vi "Channels.vi"() -> (2 "Names":string[](array[string]), 3 "Channels to Create":T1[](array[typedef]) {"Custom Config Data" format="%x"})   [LabVIEW 2021, in "TemplateCommon.lvlib"]
uses:
  TemplateCommon.lvlib
  CIF-LVCore/src/Channels/ChannelRegistrar/typedef/Channel Definition.ctl
  <vilib>/CIF Foundation/CIF Channels Core/CIFChannels/Typedef/Direction.ctl
  CIF-LVCore/src/Channels/ChannelRegistrar/typedef/Registered Channel Types.ctl
  CIF-LVCore/src/Channels/ChannelRegistrar/ChannelRegistrar.lvlib
  <vilib>/CIF Foundation/CIF Channels Core/CIFChannels/CIFChannels.lvclass
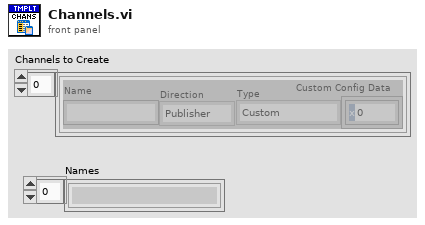
[diagram p1: front panel]
types:
  T1 = typedef "ChannelRegistrar.lvlib/Channel Definition.ctl" = cluster{"Name":string, "Direction":T2, "Type":T3, "Custom Config Data":u8[]}
  T2 = typedef "CIFChannels.lvclass/Direction.ctl" = enum16{"Publisher", "Subscriber"}
  T3 = typedef "ChannelRegistrar.lvlib/Registered Channel Types.ctl" = enum16{"Custom", "Double_Tag_CIPC", "I64_Tag_CIPC", "U64_Tag_CIPC", "U8_FIFO_CIPC", "CAN_FIFO_CIPC", "L2Enet_FIFO_CIPC", "DAQ_FIFO_CIPC", "Universal_FIFO_CIPC", "CIF_NIChn_Double", "CIF_NIChn_I64", "CIF_NIChn_U64", "CIF_NIChn_Raw", "CIF_NIChn_CAN", "CIF_NIChn_L2Enet", "CIF_NIChn_DAQ"}
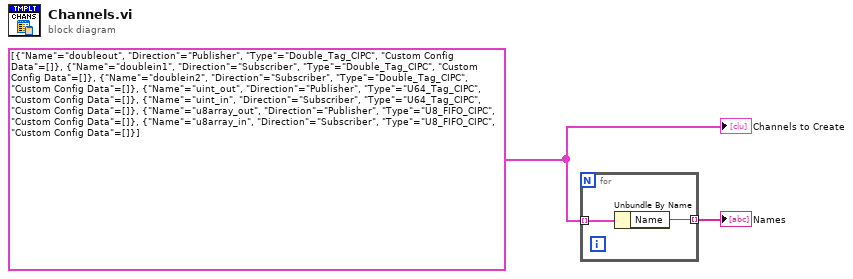
[diagram p0: block diagram]
diagram:
  w1 = T1[] [{"Name"="doubleout", "Direction"=enum."Publisher", "Type"=enum."Double_Tag_CIPC", "Custom Config Data"=[]}, {"Name"="doublein1", "Direction"=enum."Subscriber", "Type"=enum."Double_Tag_CIPC", "Custom Config Data"=[]}, {"Name"="doublein2", "Direction"=enum."Subscriber", "Type"=enum."Double_Tag_CIPC", "Custom Config Data"=[]}, {"Name"="uint_out", "Direction"=enum."Publisher", "Type"=enum."U64_Tag_CIPC", "Custom Config Data"=[]}, {"Name"="uint_in", "Direction"=enum."Subscriber", "Type"=enum."U64_Tag_CIPC", "Custom Config Data"=[]}, {"Name"="u8array_out", "Direction"=enum."Publisher", "Type"=enum."U8_FIFO_CIPC", "Custom Config Data"=[]}, {"Name"="u8array_in", "Direction"=enum."Subscriber", "Type"=enum."U8_FIFO_CIPC", "Custom Config Data"=[]}] ("Channels to Create in")
  n1 = for {
    tunnel: w1 -> [w4] mode=indexing
    tunnel: [w3] -> w2 mode=indexing
    n2 = Unbundle By Name(w4) -> ("Name"=w3:string)
  }
  "Names" <- w2
  "Channels to Create" <- w1
